vi "NXT_Motor.vi"(0 "Sequence Flow in":T4, 1 "Goal Type":T5=1 items=["Unlimited", "Distance", "Time", "Stop"], 2 "Goal (ms or degrees)":u32=360, 3 "Direction (T: Fwd)":bool=TRUE, 5 "Output (Port A)":T3 items=["Port A", "Port B", "Port C"], 7 "Power":i32=75 caption="Power (75)", 9 "Ramp Mode":T2 caption="Ramp Mode (Constant)" items=["Constant", "Ramp Up", "Ramp Down"], 12 "Stop After? (T)":bool=TRUE, 13 "Wait Until Done? (T)":bool=TRUE, 14 "Speed Regulation (F)":bool) -> (4 "Sequence Flow out":T4, 6 "Output dup":T3 items=["Port A", "Port B", "Port C"], 10 "Direction out":bool, 15 "Degrees out":i32)   [LabVIEW 2009]
doc: "Run a motor for either a specified distance, time, or unlimited duration."
uses:
  <vilib>/NXT/Block Support/NXT_OutputPort.ctl
  <vilib>/NXT/Block Support/NXT_OutputGoalType.ctl
  C:/Program Files/National Instruments/LabVIEW 2009/Targets/NI/NXT/NXTToolkit/NXT Controls/SequenceBoolean.ctl
  <vilib>/NXT/Block Support/NXT_Motor.Action.ctl
  NXTOutputRefnum.ctl
  C:/Program Files/National Instruments/LabVIEW 2009/resource/objmgr/NXTInputOutput.rc
panel:
  in  "Generic Refnum Name":T1
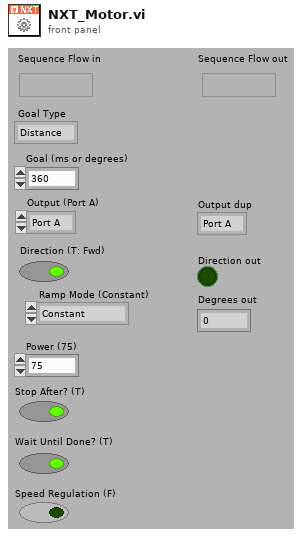
[diagram p1: front panel]
types:
  T1 = typedef "NXTOutputRefnum.ctl" = refnum<k21>
  T2 = typedef "NXT_Motor.Action.ctl" = u16
  T3 = typedef "NXT_OutputPort.ctl" = u8
  T4 = typedef "SequenceBoolean.ctl" = bool
  T5 = typedef "NXT_OutputGoalType.ctl" = u16
  T6 = typedef "MotorStageDefinition.ctl" = cluster{"Power":i8, "Mode":u8, "RegMode":T7, "RunState":T8, "Goal Type":T5, "Goal":u32, "Update Flags":u8}
  T7 = typedef "RegMode.ctl" = u8
  T8 = typedef "RunState.ctl" = u8
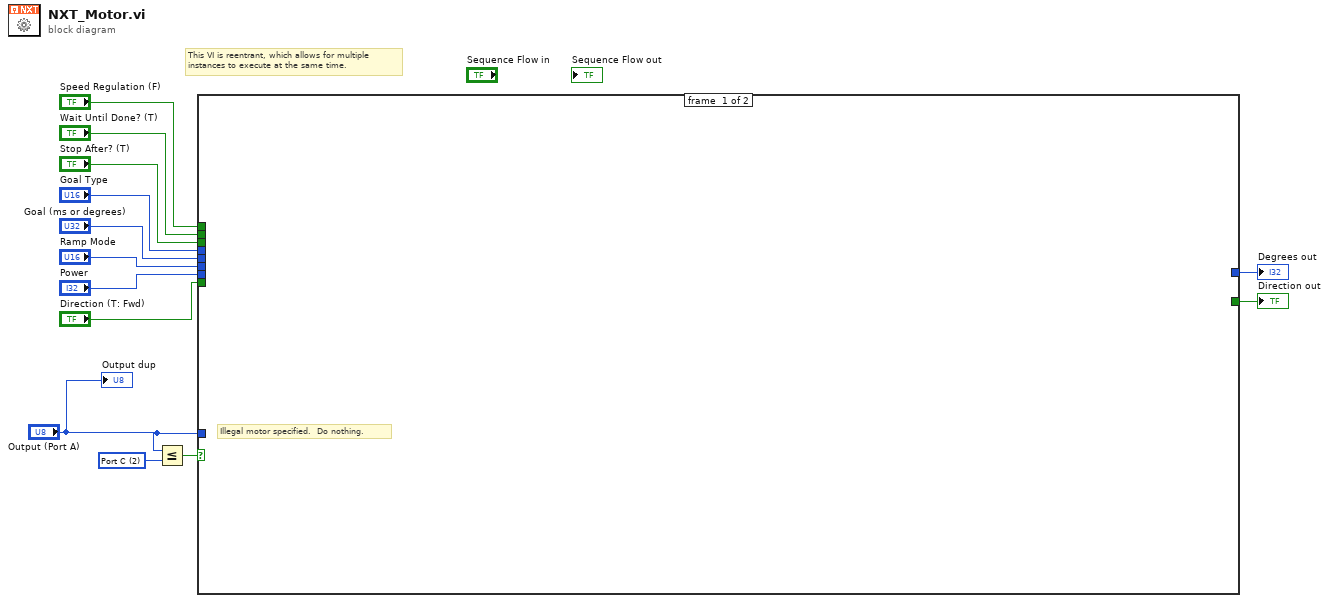
[diagram p0: block diagram]
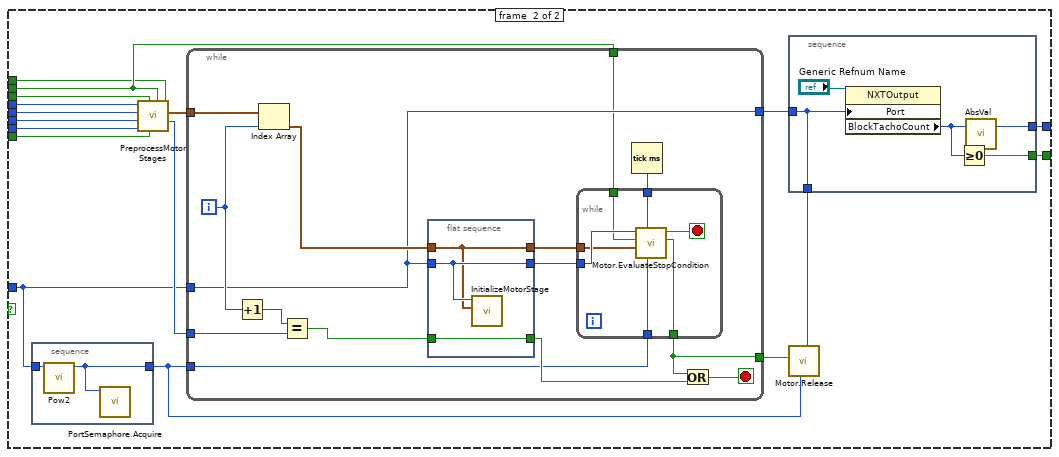
[diagram p2: hidden frame]
diagram:
  w1 = T3 2 items=["Port A", "Port B", "Port C"] ("y")
  # "This VI is reentrant, which allows for multiple\ninstances to execute at the same time."
  n1 = Less Or Equal?(x="Output (Port A)", y=w1) -> (x <= y?=w13:bool)
  n2 = case shown="True" w13 {
    tunnel: "Output (Port A)" -> [_ w26]
    tunnel: [_ w28] -> w12
    tunnel: [_ w27] -> w11
    tunnel: "Wait Until Done? (T)" -> [_ w15]
    tunnel: "Goal (ms or degrees)" -> [_ w18]
    tunnel: "Goal Type" -> [_ w17]
    tunnel: "Direction (T: Fwd)" -> [_ w21]
    tunnel: "Ramp Mode" -> [_ w19]
    tunnel: "Power" -> [_ w20]
    tunnel: "Stop After? (T)" -> [_ w16]
    tunnel: "Speed Regulation (F)" -> [_ w14]
    frame #0 {
      # "Illegal motor specified.  Do nothing."
    }
    frame #1 {
      n3 = stacked-sequence {
        tunnel: w26 -> [w37]
        tunnel: [w36] -> w24
        frame #0 {
          n4 = call <vilib>:"Pow2.vi"("Number"=w37) -> ("Pow2"=w36:u8)  [unwired: 6 in]
          n5 = call <vilib>:"PortSemaphore.Acquire.vi"("MotorBits"=w36) -> ()  [unwired: 10 in, 1 out]
        }
      }
      n6 = call "PreprocessMotorStages.vi"("Speed Regulation"=w14, "Wait"=w15, "Direction (T: Fwd)"=w21, "Stop After"=w16, "Power"=w20, "Ramp Mode"=w19, "Goal"=w18, "Goal Type"=w17) -> ("stages"=w29:i32, "stage definitions"=w30:T6[])  [unwired: 2 in]
      n7 = while {
        tunnel: w30 -> [w52]
        tunnel: w29 -> [w49]
        tunnel: w26 -> [w46]
        tunnel: w15 -> [w42]
        tunnel: [w46] -> w23
        tunnel: w24 -> [w40]
        tunnel: [w38] -> w25
        i -> [w50]
        stop <- w39 stop-if-true
        n8 = Increment(x=w50) -> (x+1=w51:i32)
        n9 = Index Array(array=w52, index=w50) -> (element=w48:T6)
        n10 = Equal?(x=w51, y=w49) -> (x = y?=w47:bool)
        n11 = flat-sequence {
          tunnel: w46 -> [w62]
          tunnel: [w62] -> w45
          tunnel: w48 -> [w60]
          tunnel: w47 -> [w61]
          tunnel: [w61] -> w41
          tunnel: [w60] -> w44
          frame #0 {
            n12 = call "InitializeMotorStage.vi"("params"=w60, "Port"=w62) -> ()  [unwired: 8 in]
          }
        }
        n13 = Tick Count (ms)() -> (millisecond timer value=w43:u32)
        n14 = while {
          tunnel: w45 -> [w59]
          tunnel: w44 -> [w58]
          tunnel: w43 -> [w57]
          tunnel: w42 -> [w56]
          tunnel: [w54] -> w38
          tunnel: w40 -> [w53]
          stop <- w55 stop-if-true
          n15 = call "Motor.EvaluateStopCondition.vi"("MotorBits"=w53, "Start Time"=w57, "StageDefinition"=w58, "Wait?"=w56, "Motor"=w59) -> ("Canceled?"=w54:bool, "Finished?"=w55:bool)  [unwired: 5 in]
        }
        n16 = Or(x=w38, y=w41) -> (x .or. y?=w39:bool)
      }
      n17 = stacked-sequence {
        tunnel: [w34] -> w28
        tunnel: [w33] -> w27
        tunnel: w23 -> [w32]
        tunnel: [w32] -> w22
        frame #0 {
          n18 = property class="NXTOutput"(reference="Generic Refnum Name", "Port"=w32) -> ("BlockTachoCount"=w35:i32)  [unwired: 1 in, 2 out]
          n19 = Greater Or Equal To 0?(x=w35) -> (x >= 0?=w33:bool)
          n20 = call <vilib>:"AbsVal.vi"("Integer"=w35) -> ("Absolute Value"=w34:i32)  [unwired: 2 in]
        }
      }
      n21 = call "Motor.Release.vi"("Motor"=w22, "MotorBits"=w24, "Cancelled?"=w25) -> ()  [unwired: 9 in]
    }
  }
  "Degrees out" <- w12
  "Direction out" <- w11
  "Output dup" <- "Output (Port A)"
